vi "字符串与路径.vi"() -> ()   [LabVIEW 2023]
panel:
  out "*(type *) &x":string
  in  "Numeric":u8
  out "string 6":string
  in  "Array":i8[](array[numeric])
  out "unsigned byte array":u8[](array[numeric])
  in  "string 5":string
  in  "replace string (\"\")":string
  out "result string 2":string
  in  "search string":string
  in  "input string":string
  out "result string":string
  out "replaced substring":string
  in  "main string length to be replaced (len. of substring)":i32
  in  "replace from main string offset (0) 2":i32
  in  "substring (\"\")":string
  in  "string 4":string
  out "substring":string
  in  "length (rest)":i32
  in  "offset (0)":i32
  in  "string 3":string
  in  "string 2":string
  out "concatenated string":string
  in  "string":string
  out "length":i32
  in  "String":string
  # "字符串 与路径 数据"
  # "Length Function"
  # "combine function"
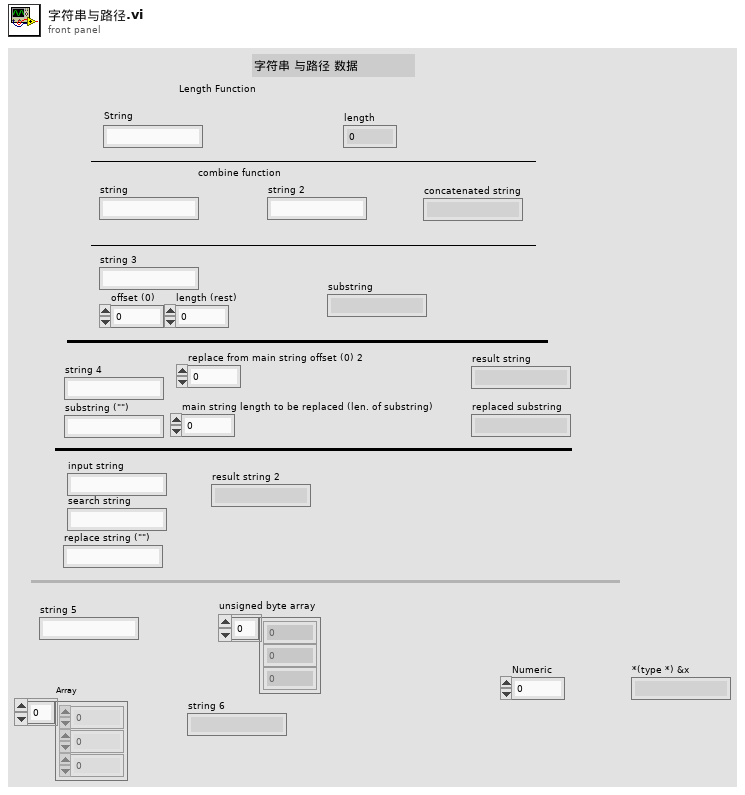
[diagram p1: front panel]
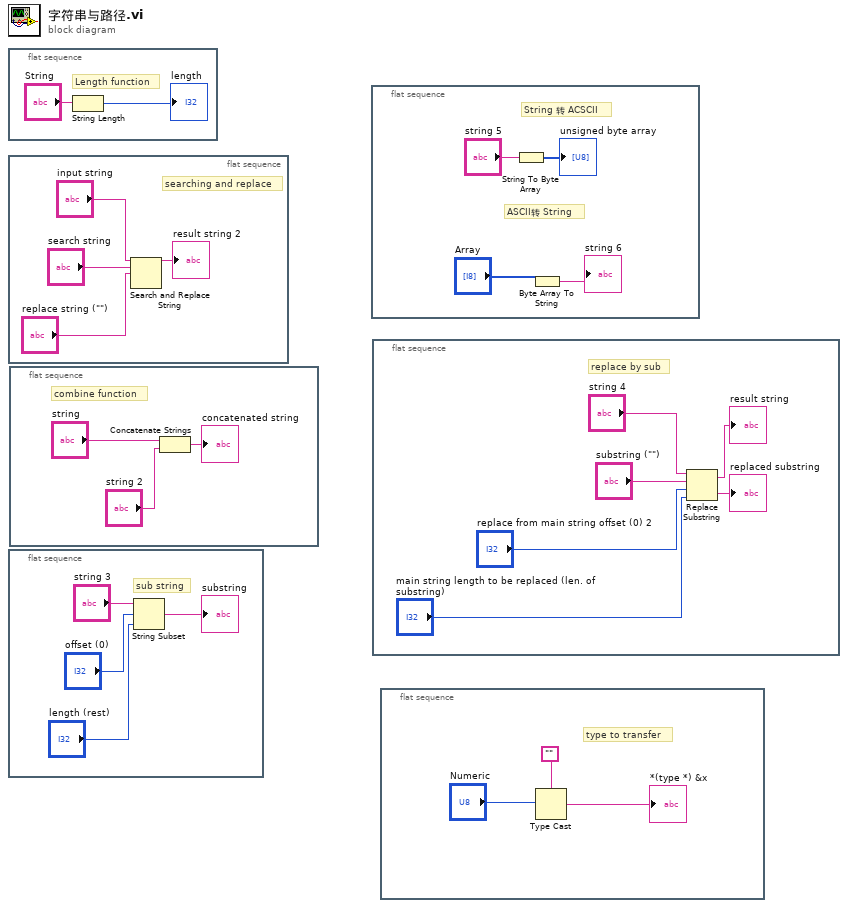
[diagram p0: block diagram]
diagram:
  n1 = flat-sequence {
    frame #0 {
      # "Length function"
      n2 = String Length(string="String") -> (length=→"length":i32)
    }
  }
  n3 = flat-sequence {
    frame #0 {
      # "searching and replace"
      n4 = Search and Replace String(input string="input string", search string="search string", replace string="replace string (\"\")") -> (result string=→"result string 2":string)  [unwired: 5 in, 3 out]
    }
  }
  n5 = flat-sequence {
    frame #0 {
      # "sub string"
      n6 = String Subset(string="string 3", offset (0)="offset (0)", length (rest)="length (rest)") -> (substring=→"substring":string)
    }
  }
  n7 = flat-sequence {
    frame #0 {
      # "combine function"
      n8 = Concatenate Strings("string", "string 2") -> (→"concatenated string":string)
    }
  }
  n9 = flat-sequence {
    frame #0 {
      # "ASCII转 String"
      # "String 转 ACSCII"
      n10 = String To Byte Array(string="string 5") -> (unsigned byte array=→"unsigned byte array":u8[])
      n11 = Byte Array To String(unsigned byte array="Array") -> (string=→"string 6":string)
    }
  }
  n12 = flat-sequence {
    frame #0 {
      # "replace by sub"
      n13 = Replace Substring(2:"main string length to be replaced (len. of substring)", 3:"replace from main string offset (0) 2", 4:"substring (\"\")", 5:"string 4") -> (0:→"replaced substring":string, 1:→"result string":string)
    }
  }
  n14 = flat-sequence {
    frame #0 {
      # "type to transfer"
      n15 = Type Cast(type="", x="Numeric") -> (*(type *) &x=→"*(type *) &x":string)
    }
  }
